vi "Set Image from File.vi"(8 "error in (no error)":errorcluster, 9 "State":T1, 10 "path":path, 11 "Button in":refnum<class "Button.lvclass">) -> (0 "error out":errorcluster, 3 "Button out":refnum<class "Button.lvclass">)   [LabVIEW 2018, in "Button.lvclass"]
doc: "Sets the button images by loading a picture (bmp/png/jpeg) from a file"
uses:
  Button.lvclass
  <userlib>/_OpenG.lib/file/file.llb/Strip Path Extension - Path__ogtk.vi
  Type Defs/Button Status.ctl
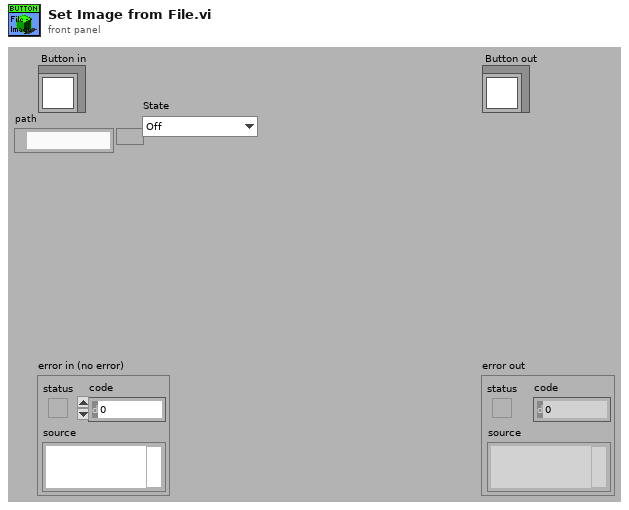
[diagram p1: front panel]
types:
  T1 = typedef "Button.lvclass/Button Status.ctl" = enum16{"Off", "Hover", "On", "Disabled"}
  T2 = typedef "imagedata.ctl" = cluster{"image type":i32, "image depth":i32, "image":u8[], "mask":u8[], "colors":u32[], "Rectangle":cluster{"left":i16, "top":i16, "right":i16, "bottom":i16}}
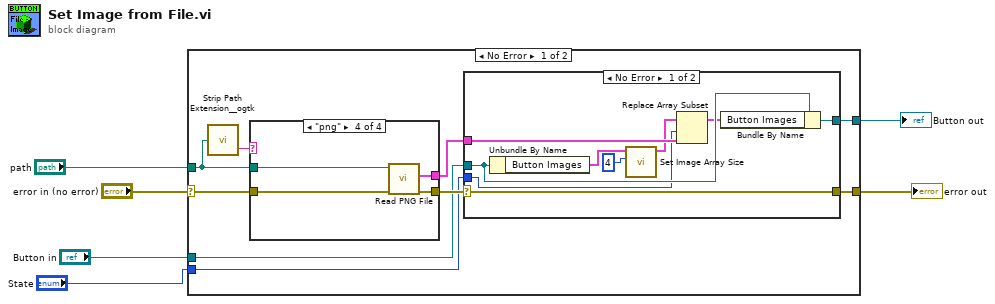
[diagram p0: block diagram]
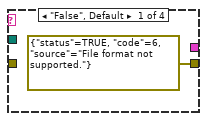
[diagram p3: hidden frame]
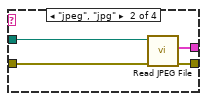
[diagram p4: hidden frame]
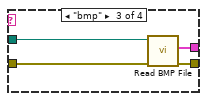
[diagram p5: hidden frame]
diagram:
  n1 = case shown="No Error" "error in (no error)" {
    selector: "error in (no error)" -> [w12 w41]
    tunnel: [w7 w41] -> w5
    tunnel: [w8 w40] -> w3
    tunnel: "Button in" -> [w9 w40]
    tunnel: "path" -> [w11 _]
    tunnel: "State" -> [w10 _]
    frame No Error {
      n2 = call-poly <userlib>:"Strip Path Extension__ogtk.vi"("path"=w11) -> ("extension"=w15:string)  [unwired: 1 out]
      n3 = case shown="\"png\"" w15 {
        tunnel: w11 -> [_ w30 w34 w38]
        tunnel: w12 -> [_ w31 w35 w39]
        tunnel: [_ w29 w32 w36] -> w14
        tunnel: [errorcluster {"status"=TRUE, "code"=6, "source"="File format not supported."} ("error out") w28 w33 w37] -> w13
        frame "False", Default {
        }
        frame "jpeg", "jpg" {
          n4 = call <vilib>:"Read JPEG File.vi"("error in (no error)"=w31, "path to JPEG file"=w30) -> ("error out"=w28:errorcluster, "image data"=w29:T2)  [unwired: 8 out]
        }
        frame "bmp" {
          n5 = call <vilib>:"Read BMP File.vi"("error in (no error)"=w35, "path to BMP file"=w34) -> ("error out"=w33:errorcluster, "image data"=w32:T2)  [unwired: 8 out]
        }
        frame "png" {
          n6 = call <vilib>:"Read PNG File.vi"("error in (no error)"=w39, "path to PNG file"=w38) -> ("error out"=w37:errorcluster, "image data"=w36:T2)  [unwired: 8 out]
        }
      }
      n7 = case shown="No Error" w13 {
        selector: w13 -> [w24 w26]
        tunnel: w14 -> [w20 _]
        tunnel: w10 -> [w19 _]
        tunnel: w9 -> [w23 w25]
        tunnel: [w21 w25] -> w8
        tunnel: [w24 w26] -> w7
        frame No Error {
          n8 = Unbundle By Name(w23) -> ("Button Images"=w18:T2[])
          n9 = call "Set Image Array Size.vi"("Buttons Displayed"=4, "Button Images in"=w18) -> ("Button Images out"=w17:T2[])  [unwired: 9 in]
          n10 = Replace Array Subset(array=w17, new element=w20, index=w19) -> (w22:T2[])
          n11 = Bundle By Name(cluster=w23, "Button Images"=w22) -> (w21:refnum<class "Button.lvclass">)
        }
        frame Error {
        }
      }
    }
    frame Error {
    }
  }
  "error out" <- w5
  "Button out" <- w3
